vi "HistogramManual2003.vi"   [LabVIEW 2013]
uses:
  <vilib>/Heliosphere Research LLC/Advanced Plotting Toolkit/api_plotting/Histogram_Manual.vi
  <vilib>/Heliosphere Research LLC/Advanced Plotting Toolkit/Advanced Plotting Toolkit.lvlib
types:
  T1 = typedef "Advanced Plotting Toolkit.lvlib/PlotID.ctl" = i32
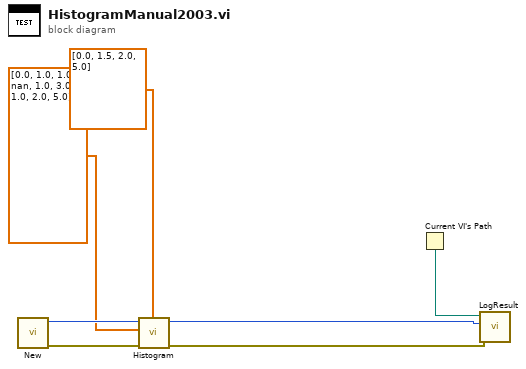
[diagram p0: block diagram]
diagram:
  n1 = call <vilib>:"New.vi"() -> ("error out"=w4:errorcluster, "Plot ID"=w7:T1)  [unwired: 10 in]
  n2 = call-poly <vilib>:"Histogram.vi"("Bins"=dbl[] [0.0, 1.5, 2.0, 5.0], "error in (no error)"=w4, "Data"=dbl[] [0.0, 1.0, 1.0, nan, 1.0, 3.0, 1.0, 2.0, 5.0], "Plot ID"=w7) -> ("error out"=w3:errorcluster, "Plot ID Out"=w6:T1)  [unwired: 6 in]
  n3 = Current VI's Path() -> (path=w5:path)
  n4 = call "LogResult.vi"("Test Result"=w3, "Test Artifact"=w6, "VI Path"=w5) -> ()  [unwired: 9 in]
